vi "Execute.vi"(8 "error in (no error)":errorcluster, 9 "System in":refnum<class "System.lvclass">, 10 "Command in":refnum<class "Command.lvclass">, 11 "Grabber-ExtendedState in":refnum<class "GrabberArms-ExtendedState.lvclass">) -> (0 "error out":errorcluster, 2 "Next State":refnum<class "State.lvclass">, 3 "Grabber-ExtendedState out":refnum<class "GrabberArms-ExtendedState.lvclass">)   [LabVIEW 2013, in "GrabberArms-ExtendedState.lvclass"]
uses:
  GrabberArms-ExtendedState.lvclass
  Commands/Command/Command.lvclass
  Systems/System/System.lvclass
  State/State.lvclass
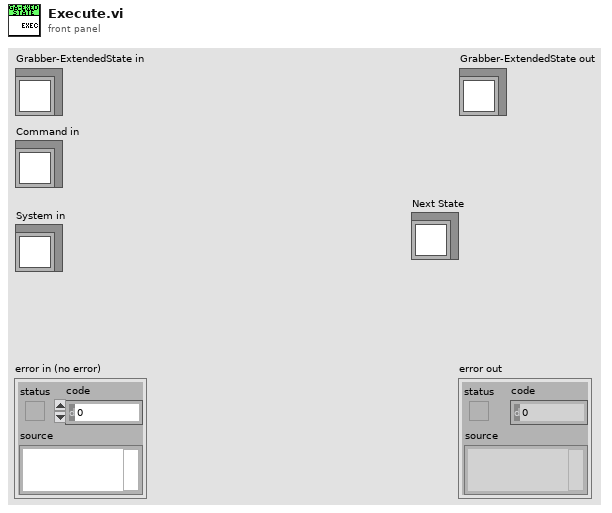
[diagram p1: front panel]
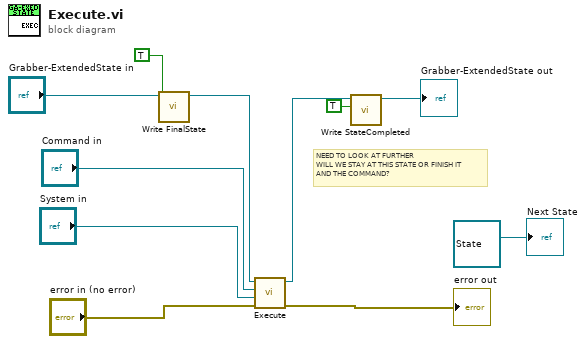
[diagram p0: block diagram]
diagram:
  # "NEED TO LOOK AT FURTHER\nWILL WE STAY AT THIS STATE OR FINISH IT \nAND THE COMMAND?"
  n1 = call-dynamic "Write FinalState.vi"("FinalState"=TRUE, "State in"="Grabber-ExtendedState in") -> ("State out"=w4:refnum<class "GrabberArms-ExtendedState.lvclass">)  [unwired: 8 in, 1 out]
  n2 = call-parent "Execute.vi"("error in (no error)"="error in (no error)", "System in"="System in", "Command in"="Command in", "State in"=w4) -> ("error out"=→"error out":errorcluster, "State out"=w10:refnum<class "GrabberArms-ExtendedState.lvclass">)  [unwired: 5 in, 1 out]
  n3 = call-dynamic "Write StateCompleted.vi"("StateCompleted"=TRUE, "State in"=w10) -> ("State out"=→"Grabber-ExtendedState out":refnum<class "GrabberArms-ExtendedState.lvclass">)  [unwired: 8 in, 1 out]
  "Next State" <- refnum<class "State.lvclass"> refnum ("State.lvclass")
